vi "다양한연산.vi"() -> ()   [LabVIEW 2019]
panel:
  in  "열거형":enum16{"더하기", "빼기", "곱하기", "나누기", "최대/최소"}(ring)
  out "결과 2":dbl
  out "결과":dbl
  in  "B":dbl
  in  "A":dbl
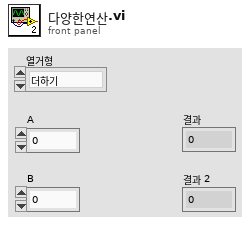
[diagram p1: front panel]
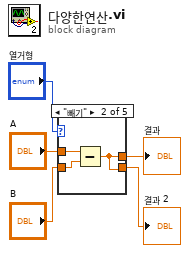
[diagram p0: block diagram]
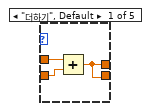
[diagram p2: hidden frame]
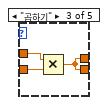
[diagram p3: hidden frame]
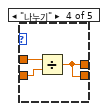
[diagram p4: hidden frame]
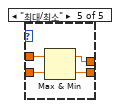
[diagram p5: hidden frame]
diagram:
  n1 = case shown="\"빼기\"" "열거형" {
    tunnel: "B" -> [w8 w11 w14 w17 w21]
    tunnel: "A" -> [w7 w10 w13 w16 w20]
    tunnel: [w6 w9 w12 w15 w19] -> w3
    tunnel: [w6 w9 w12 w15 w18] -> w1
    frame "더하기", Default {
      n2 = Add(x=w7, y=w8) -> (x+y=w6:dbl)
    }
    frame "빼기" {
      n3 = Subtract(x=w10, y=w11) -> (x-y=w9:dbl)
    }
    frame "곱하기" {
      n4 = Multiply(x=w13, y=w14) -> (x*y=w12:dbl)
    }
    frame "나누기" {
      n5 = Divide(x=w16, y=w17) -> (x/y=w15:dbl)
    }
    frame "최대/최소" {
      n6 = Max & Min(x=w20, y=w21) -> (max(x,y)=w19:dbl, min(x,y)=w18:dbl)
    }
  }
  "결과" <- w3
  "결과 2" <- w1
